vi "NTV_Spare 1 Status.vi"(7 "Read(f) Write(t)":bool, 11 "Shooter Speed":T1) -> (3 "Shooter Speed":T1)   [LabVIEW 2023]
uses:
  TypeDefs/Cluster_Shooter Speed Data.ctl
  <vilib>/Rock Robotics/Network Tables/NT Read Numeric Array.vi
  <vilib>/Rock Robotics/Network Tables/NT Write Numeric Array.vi
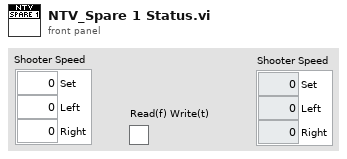
[diagram p1: front panel]
types:
  T1 = typedef "Cluster_Shooter Speed Data.ctl" = cluster{"Set":dbl, "Left":dbl, "Right":dbl}
  T2 = cluster{"value[0]":dbl, "value[1]":dbl, "value[2]":dbl}
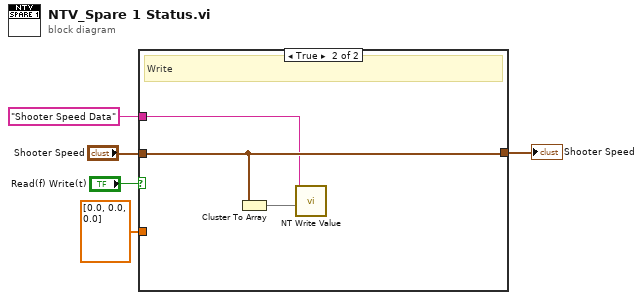
[diagram p0: block diagram]
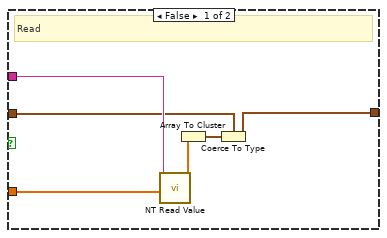
[diagram p2: hidden frame]
diagram:
  n1 = case shown="True" "Read(f) Write(t)" {
    tunnel: "Shooter Speed" -> [w7 w14]
    tunnel: "Shooter Speed Data" ("Name") -> [w11 w12]
    tunnel: [w8 w14] -> w2
    tunnel: dbl[] [0.0, 0.0, 0.0] ("Default Value") -> [w6 _]
    frame False {
      # "Read"
      n2 = call-poly <vilib>:"NT Read Value.vi"("default value"=w6, "name"=w11) -> ("value"=w10:dbl[])  [unwired: 7 in, 2 out]
      n3 = Array To Cluster(array=w10) -> (cluster=w9:T2)
      n4 = Coerce To Type(0:w9, 1:w7) -> (2:w8:T1)
    }
    frame True {
      # "Write"
      n5 = Cluster To Array(cluster=w14) -> (array=w13:dbl[])
      n6 = call-poly <vilib>:"NT Write Value.vi"("value"=w13, "name"=w12) -> ()  [unwired: 9 in, 1 out]
    }
  }
  "Shooter Speed" <- w2
